vi "Get Data.vi"(8 "error in":errorcluster, 11 "Cfg Dev in":refnum<class "Vaisala.lvclass">) -> (0 "error out":errorcluster, 2 "Data":refnum<class "Data.lvclass">, 3 "Cfg Dev out":refnum<class "Vaisala.lvclass">)   [LabVIEW 2014, in "Vaisala Library.lvlib" / "Vaisala.lvclass"]
uses:
  Vaisala.lvclass
  reusable/Data/Data.lvclass
  reusable/Session APIs/Serial/Serial Session.lvclass
  Data/Vaisala Data.lvclass
  Configurable Device/Configurable Device.lvclass/Configurable Device.ctl
  reusable/Data/Data.lvclass/Data.ctl
  Vaisala.lvclass/Vaisala.ctl
  Data/Vaisala Data.lvclass/Vaisala Data.ctl
  Configurable Device/Read ID.vi
  Configurable Device/Read Log Session.vi
  Data/Write T.vi
  Data/Write RH.vi
  Data/Write Td.vi
  reusable/Data/Write write time.vi
  reusable/Session APIs/Serial/Public/Get Data/Get String.vi
  reusable/Data/Write measTime.vi
  <userlib>/_Session Fwk/Session - Root.lvclass
  reusable/Session APIs/Session Log/System Log.lvclass
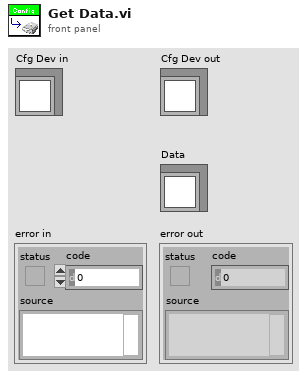
[diagram p1: front panel]
types:
  T1 = typedef "Session - Root.lvclass/Session Handle.ctl" = refnum<data-value>
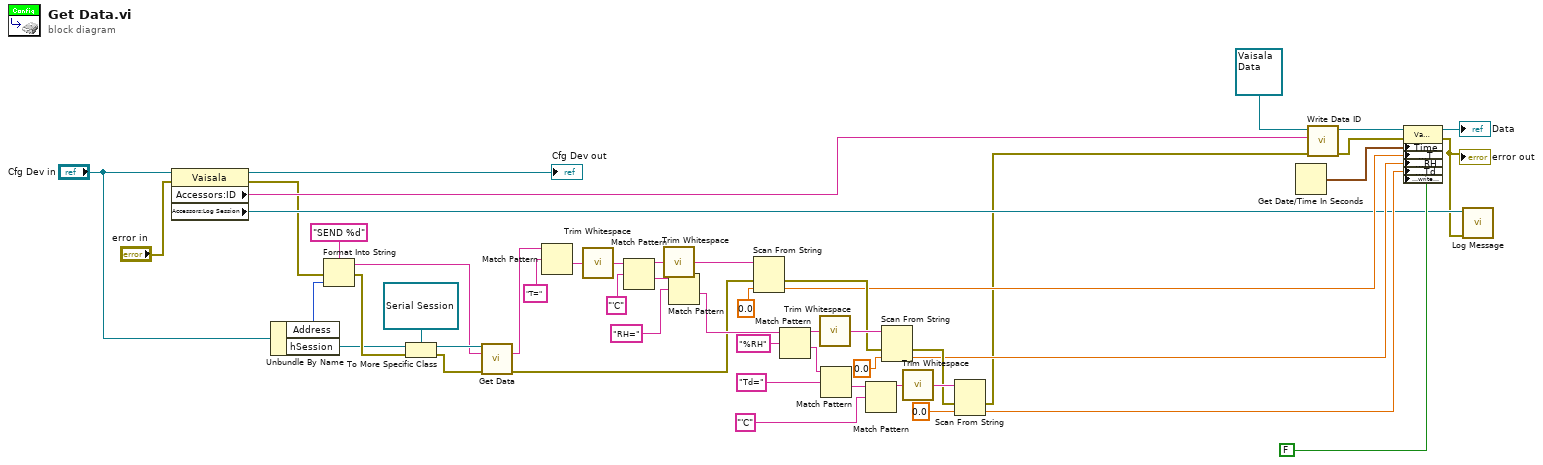
[diagram p0: block diagram]
diagram:
  n1 = property class="Vaisala"(reference="Cfg Dev in", error in="error in") -> (reference out=→"Cfg Dev out":refnum<class "Vaisala.lvclass">, error out=w3:errorcluster, "Accessors:ID"=w12:string, "Accessors:Log Session"=w8:T1)
  n2 = Unbundle By Name("Cfg Dev in") -> ("Address"=w50:u8, "hSession"=w22:T1)
  n3 = Format Into String(format string="SEND %d", error in=w3, w50) -> (resulting string=w17:string, error out=w23:errorcluster)  [unwired: 1 in]
  n4 = To More Specific Class(target class=refnum<data-value> refnum ("hSession"), reference=w22, error in=w23) -> (specific class reference=w20:refnum<data-value>, error out=w19:errorcluster)
  n5 = call-poly "Get Data.vi"("Session Handle in"=w20, "CMD"=w17, "error in"=w19) -> ("DataOut"=w18:string, "error out"=w2:errorcluster)  [unwired: 10 in, 1 out]
  n6 = Match Pattern(string=w18, regular expression="T=") -> (after substring=w47:string)  [unwired: 1 in, 3 out]
  n7 = call <vilib>:"Trim Whitespace.vi"("string"=w47) -> ("trimmed string"=w46:string)  [unwired: 1 in]
  n8 = Match Pattern(string=w46, regular expression="'C") -> (before substring=w44:string, after substring=w41:string)  [unwired: 1 in, 2 out]
  n9 = call <vilib>:"Trim Whitespace.vi"("string"=w44) -> ("trimmed string"=w43:string)  [unwired: 1 in]
  n10 = Match Pattern(string=w41, regular expression="RH=") -> (after substring=w38:string)  [unwired: 1 in, 3 out]
  n11 = Scan From String(input string=w43, error in=w2, default 1=sgl 0.0 ("output 1")) -> (error out=w27:errorcluster, output 1=w14:sgl)  [unwired: 2 in, 2 out]
  n12 = Match Pattern(string=w38, regular expression="%RH") -> (before substring=w35:string, after substring=w33:string)  [unwired: 1 in, 2 out]
  n13 = call <vilib>:"Trim Whitespace.vi"("string"=w35) -> ("trimmed string"=w36:string)  [unwired: 1 in]
  n14 = Match Pattern(string=w33, regular expression="Td=") -> (after substring=w31:string)  [unwired: 1 in, 3 out]
  n15 = Match Pattern(string=w31, regular expression="'C") -> (before substring=w28:string)  [unwired: 1 in, 3 out]
  n16 = Scan From String(input string=w36, error in=w27, default 1=sgl 0.0 ("output 1")) -> (error out=w26:errorcluster, output 1=w15:sgl)  [unwired: 2 in, 2 out]
  n17 = call <vilib>:"Trim Whitespace.vi"("string"=w28) -> ("trimmed string"=w29:string)  [unwired: 1 in]
  n18 = Scan From String(input string=w29, error in=w26, default 1=sgl 0.0 ("output 1")) -> (error out=w1:errorcluster, output 1=w16:sgl)  [unwired: 2 in, 2 out]
  n19 = Get Date/Time In Seconds() -> (seconds since 1Jan1904=w25:timestamp)
  n20 = call "Write Data ID.vi"("error in"=w1, "Data ID"=w12, "Data in"=refnum<class "Vaisala Data.lvclass"> refnum ("Vaisala Library.lvlib:Vaisala Data.lvclass")) -> ("error out"=w10:errorcluster, "Data out"=w11:refnum<class "Vaisala Data.lvclass">)  [unwired: 7 in]
  n21 = property class="Vaisala Data"(reference=w11, error in=w10, "Time"=w25, "Accessors:T"=w14, "Accessors:RH"=w15, "Accessors:Td"=w16, "Accessors:write time"=FALSE ("write time")) -> (reference out=→"Data":refnum<class "Vaisala Data.lvclass">, error out=w7:errorcluster)
  "error out" <- w7
  n22 = call "Log Message.vi"("error in"=w7, "session in"=w8) -> ()  [unwired: 8 in, 2 out]
